vi "Get Properties from File by Class and or ID.vi"(10 "Class ID":string, 11 "Class Name":string) -> (3 "Array":T1(array[cluster]))   [LabVIEW 2023]
doc: "Give the UNique ID or CLass Name, return the property heirarchy from the array of all LV classes.\n\nNote this will not always give the same result as getting the list of values from a property node, especially with regard to the value properties. (Is this true?)"
panel:
  out "exe time (ms)":u32
  # "OR"
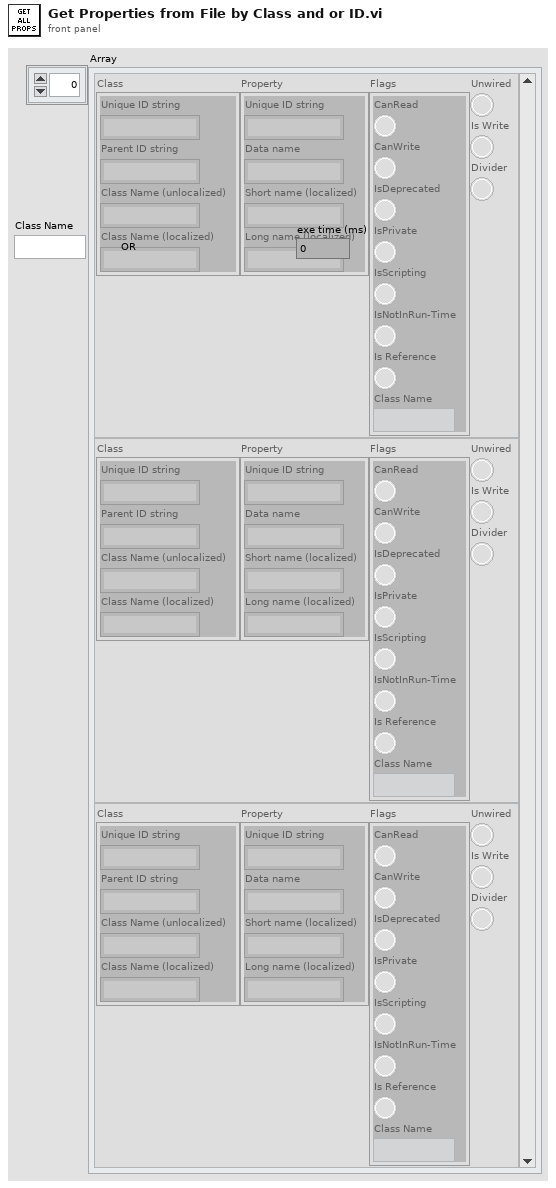
[diagram p1: front panel]
types:
  T1 = cluster{"Class":cluster{"Unique ID string":string, "Parent ID string":string, "Class Name (unlocalized)":string, "Class Name (localized)":string}, "Property":cluster{"Unique ID string":string, "Data name":string, "Short name (localized)":string, "Long name (localized)":string}, "Flags":cluster{"CanRead":bool, "CanWrite":bool, "IsDeprecated":bool, "IsPrivate":bool, "IsScripting":bool, "IsNotInRun-Time":bool, "Is Reference":bool, "Class Name":string}, "Divider":bool, "Is Write":bool, "Unwired":bool}[]
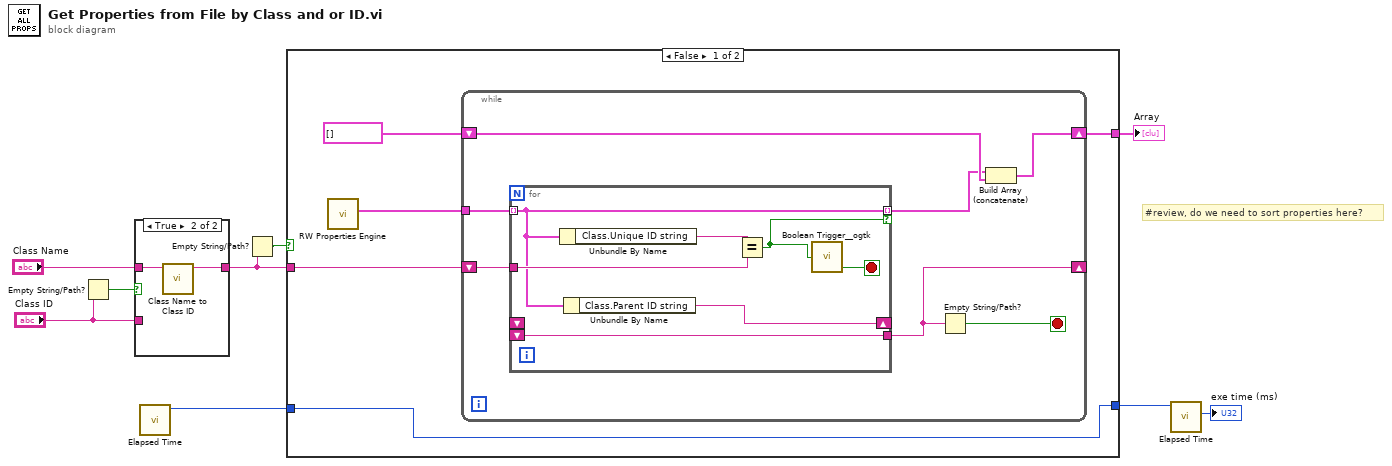
[diagram p0: block diagram]
diagram:
  # "#review, do we need to sort properties here?"
  n1 = Empty String/Path?(string/path="Class ID") -> (empty?=w7:bool)
  n2 = case shown="True" w7 {
    tunnel: "Class Name" -> [_ w12]
    tunnel: [w10 w11] -> w5
    tunnel: "Class ID" -> [w10 _]
    frame False {
    }
    frame True {
      n3 = call "Class Name to Class ID.vi"("Class Name"=w12) -> ("Class ID"=w11:string)  [unwired: 10 in]
    }
  }
  n4 = call "Elapsed Time.vi"() -> ("millisecond timer value"=w2:u32)  [unwired: 8 in, 3 out]
  n5 = Empty String/Path?(string/path=w5) -> (empty?=w4:bool)
  n6 = case shown="False" w4 {
    tunnel: [w17 _] -> w9
    tunnel: w5 -> [w15 _]
    tunnel: [w13 w32] -> w3
    tunnel: w2 -> [w13 w32]
    frame False {
      n7 = call "RW Properties Engine.vi"() -> ("Properties Out"=w14:T1)  [unwired: 7 in, 4 out]
      n8 = while {
        shift-right: [w19] -> _
        shift-left: w15 -> [w23]
        tunnel: w14 -> [w24]
        shift-right: [w20] -> w17
        shift-left: T1 [] -> [w21]
        stop <- w22 stop-if-true
        n9 = for {
          tunnel: w24 -> [w29] mode=indexing
          tunnel: w23 -> [w30]
          tunnel: [w29] -> w18 mode=indexing if=w28
          shift-right: [w26] -> _
          shift-left: _ -> [_]
          shift-left: _ -> [w25]
          tunnel: [w25] -> w19
          stop <- w27 stop-if-true
          n10 = Unbundle By Name(w29) -> ("Class.Unique ID string"=w31:string)
          n11 = Unbundle By Name(w29) -> ("Class.Parent ID string"=w26:string)
          n12 = Equal?(x=w31, y=w30) -> (x = y?=w28:bool)
          n13 = call <userlib>:"Boolean Trigger__ogtk.vi"("Boolean Input"=w28) -> ("Falling Edge"=w27:bool)  [unwired: 1 in, 1 out]
        }
        n14 = Empty String/Path?(string/path=w19) -> (empty?=w22:bool)
        n15 = Build Array (concatenate)(w18, w21) -> (w20:T1)
      }
    }
    frame True {
    }
  }
  "Array" <- w9
  n16 = call "Elapsed Time.vi"("past time"=w3) -> ("elapsed time (ms)"=→"exe time (ms)":u32)  [unwired: 7 in, 3 out]
